vi "CommandRecieve.vi"(8 "error in (no error)":errorcluster, 10 "NetworkStreamReader in":refnum<class "NetworkStreamReader.lvclass">) -> (0 "error out":errorcluster, 2 "NetworkStreamReader out":refnum<class "NetworkStreamReader.lvclass">)   [LabVIEW 2012]
doc: "Recieves the Mission data from the OCU and stroes it in the Reciecved Missions Queue\n\nElizabeth Mahon and Victoria\n01/14"
uses:
  RIO-OCU_Comm/NetworkStreams/Reader/NetworkStreamReader.lvclass
  RIO-OCU_Comm/ToRIO.ctl
  Classes/Missions/GenericMission/GenericMission.lvclass
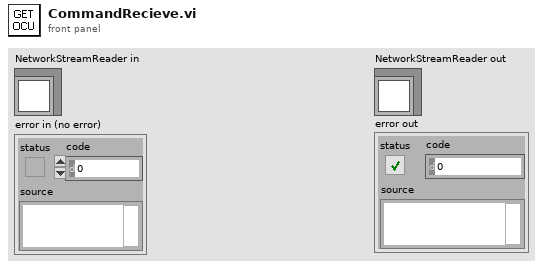
[diagram p1: front panel]
types:
  T1 = typedef "ToRIO.ctl" = cluster{"Mission":refnum<class "GenericMission.lvclass">}
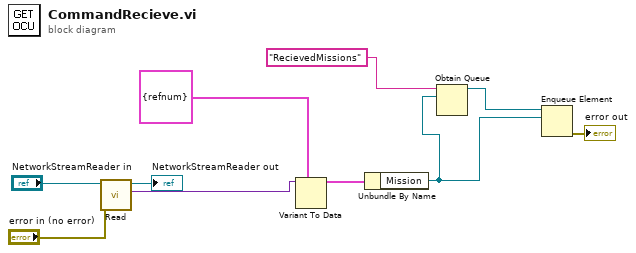
[diagram p0: block diagram]
diagram:
  n1 = call "Read.vi"("error in (no error)"="error in (no error)", "NetworkStreamReader in"="NetworkStreamReader in") -> ("element"=w3:variant, "NetworkStreamReader out"=→"NetworkStreamReader out":refnum<class "NetworkStreamReader.lvclass">)  [unwired: 5 in, 3 out]
  n2 = Variant To Data(type=T1 {"Mission"=refnum} ("To RIO"), Variant=w3) -> (data=w4:T1)  [unwired: 1 in, 1 out]
  n3 = Unbundle By Name(w4) -> ("Mission"=w8:refnum<class "GenericMission.lvclass">)
  n4 = Obtain Queue(name (unnamed)="RecievedMissions", element data type=w8) -> (queue out=w9:refnum<queue>)  [unwired: 3 in, 2 out]
  n5 = Enqueue Element(queue=w9, element=w8) -> (error out=→"error out":errorcluster)  [unwired: 2 in, 2 out]
